vi "Layer2_ReceiveResponse.vi"(8 "Error In":errorcluster, 9 "PacketNum\nWaiting Ack":u16=9915, 10 "Expecting Response":bool, 11 "Serial Port to Use":refnum<visa-resource-name>="COM8") -> (0 "Layer2 Payload":string, 1 "No Errors":bool, 2 "Response Received":bool, 3 "Msg Acknowledged":bool, 4 "Error Out":errorcluster, 5 "Serial Port to Use (out)":refnum<visa-resource-name>)   [LabVIEW 2012]
uses:
  Arduino_Serial_GlobalConstants.vi
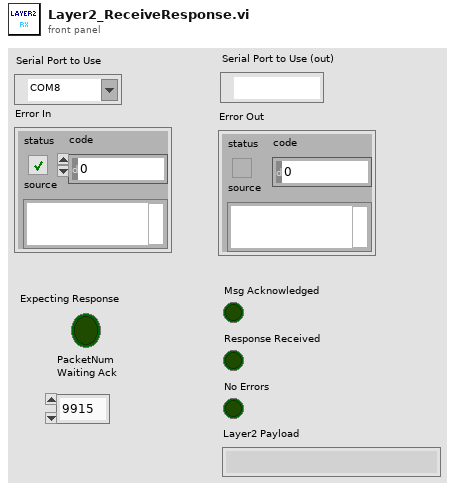
[diagram p1: front panel]
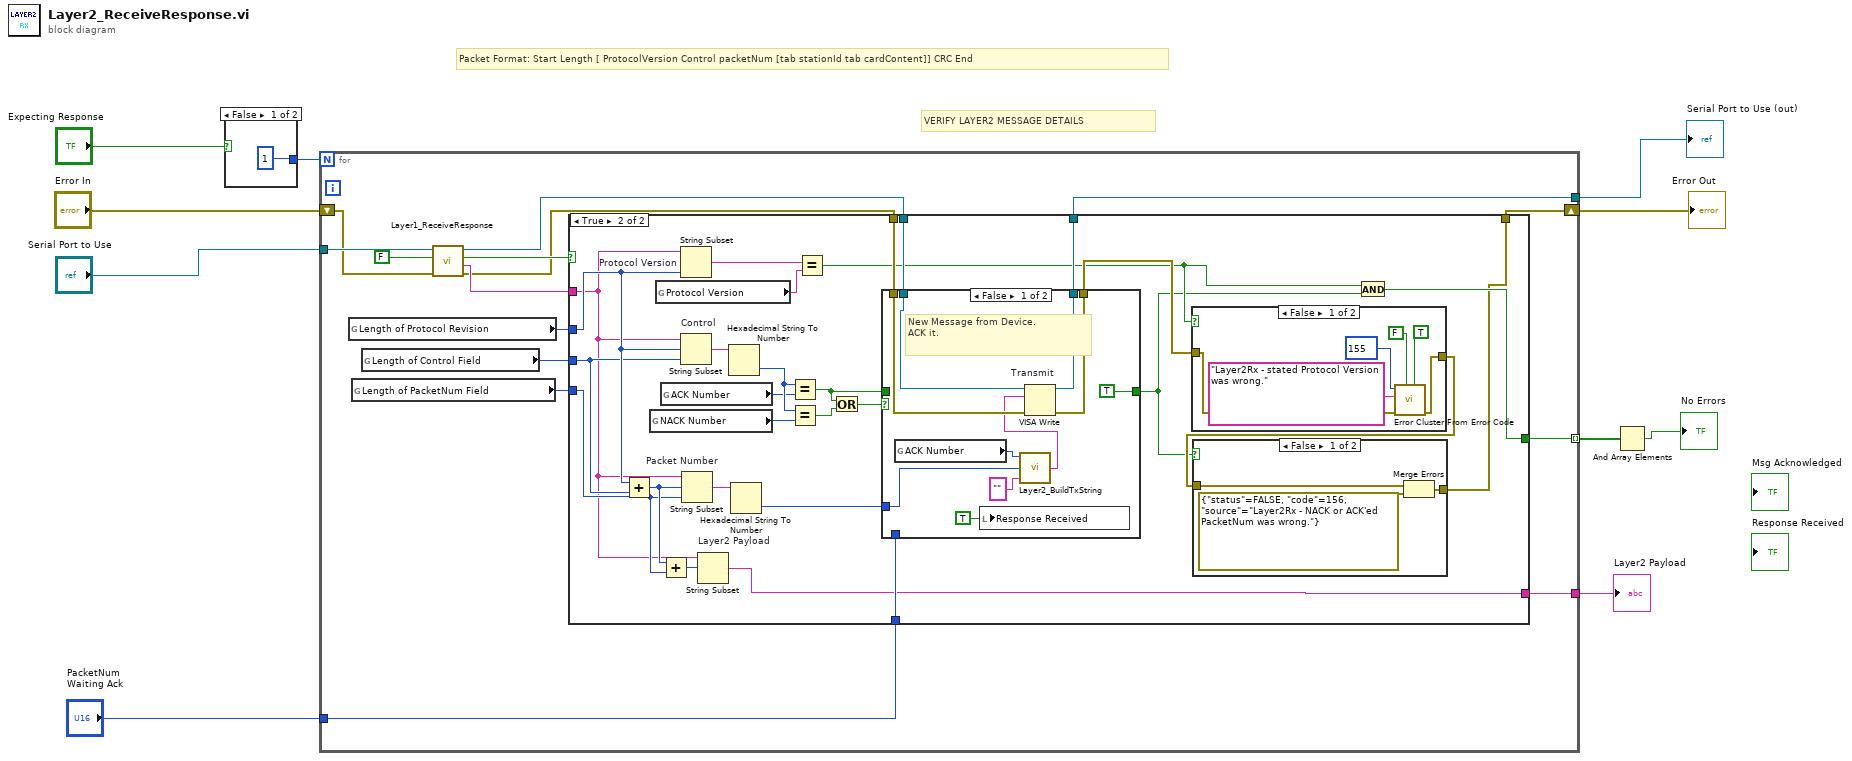
[diagram p0: block diagram]
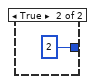
[diagram p2: hidden frame]
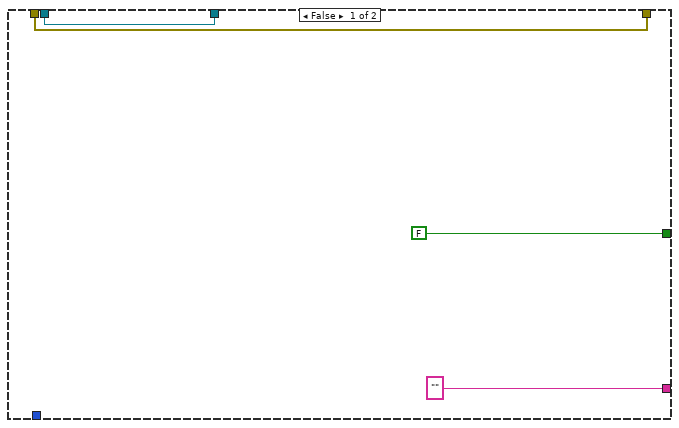
[diagram p3: hidden frame]
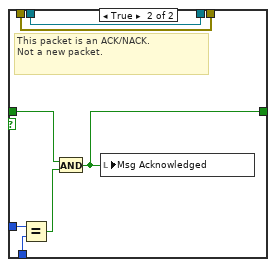
[diagram p6: hidden frame]
diagram:
  # "Packet Format: Start Length [ ProtocolVersion Control packetNum [tab stationId tab cardContent]] CRC End"
  # "VERIFY LAYER2 MESSAGE DETAILS"
  n1 = case shown="False" "Expecting Response" {
    tunnel: [1 ("Numeric") 2 ("Numeric")] -> w6
    frame False {
    }
    frame True {
    }
  }
  n2 = for {
    N: w6 -> [_]
    tunnel: "Serial Port to Use" -> [w27]
    tunnel: [w25] -> w8
    tunnel: [w24] -> w4 mode=indexing
    tunnel: "PacketNum\nWaiting Ack" -> [w23]
    shift-right: [w13] -> w1
    shift-left: "Error In" -> [w26]
    tunnel: [w14] -> w2
    n3 = global read "Arduino_Serial_GlobalConstants.vi" "Length of Protocol Revision"() -> (w20:i32)
    n4 = global read "Arduino_Serial_GlobalConstants.vi" "Length of PacketNum Field"() -> (w22:i32)
    n5 = global read "Arduino_Serial_GlobalConstants.vi" "Length of Control Field"() -> (w21:i32)
    n6 = call "Layer1_ReceiveResponse.vi"("Error In"=w26, "Close Port After?"=FALSE, "Serial Port to Use (In)"=w27) -> ("Error Out"=w15:errorcluster, "Layer1 Payload"=w18:string, "Layer 1 Valid Packet"=w17:bool, "Serial Port to Use (out)"=w16:refnum<visa-resource-name>)  [unwired: 3 in, 2 out]
    n7 = case shown="True" w17 {
      tunnel: [FALSE w37] -> w24
      tunnel: w18 -> [_ w51]
      tunnel: ["" ("read buffer") w38] -> w25
      tunnel: w23 -> [_ w41]
      tunnel: w22 -> [_ w53]
      tunnel: w21 -> [_ w56]
      tunnel: w20 -> [_ w57]
      tunnel: w15 -> [w28 w44]
      tunnel: w16 -> [w29 w43]
      tunnel: [w29 w42] -> w14
      tunnel: [w28 w34] -> w13
      frame False {
      }
      frame True {
        n8 = Add(x=w57, y=w56) -> (x+y=w54:i32)
        n9 = global read "Arduino_Serial_GlobalConstants.vi" "NACK Number"() -> (w47:i32)
        n10 = global read "Arduino_Serial_GlobalConstants.vi" "Protocol Version"() -> (w58:string)
        n11 = global read "Arduino_Serial_GlobalConstants.vi" "ACK Number"() -> (w48:i32)
        n12 = Add(x=w54, y=w53) -> (x+y=w52:i32)
        n13 = String Subset "Protocol Version"(string=w51, length (rest)=w57) -> (substring=w59:string)  [unwired: 1 in]
        n14 = String Subset "Control"(string=w51, offset (0)=w57, length (rest)=w56) -> (substring=w50:string)
        n15 = String Subset "Packet Number"(string=w51, offset (0)=w54, length (rest)=w53) -> (substring=w55:string)
        n16 = String Subset "Layer2 Payload"(string=w51, offset (0)=w52) -> (substring=w38:string)  [unwired: 1 in]
        n17 = Hexadecimal String To Number(string=w50) -> (number=w49:u32)  [unwired: 2 in, 1 out]
        n18 = Hexadecimal String To Number(string=w55) -> (number=w40:u32)  [unwired: 2 in, 1 out]
        n19 = Equal?(x=w49, y=w48) -> (x = y?=w39:bool)
        n20 = Equal?(x=w49, y=w47) -> (x = y?=w46:bool)
        n21 = Equal?(x=w59, y=w58) -> (x = y?=w35:bool)
        n22 = Or(x=w39, y=w46) -> (x .or. y?=w45:bool)
        n23 = case shown="False" w45 {
          tunnel: w44 -> [w74 w86]
          tunnel: w43 -> [w75 w87]
          tunnel: [w73 w87] -> w42
          tunnel: [w72 w86] -> w36
          tunnel: w41 -> [_ w85]
          tunnel: w40 -> [w78 w84]
          tunnel: [TRUE w81] -> w32
          tunnel: w39 -> [_ w82]
          frame False {
            # "New Message from Device.\nACK it."
            n24 = global read "Arduino_Serial_GlobalConstants.vi" "ACK Number"() -> (w76:i32)
            n25 = local write "Response Received"(TRUE ("Response Received")) -> ()
            n26 = call "Layer2_BuildTxString.vi"("Message"="", "PacketNum"=w78, "Control"=w76) -> ("Write Buffer"=w71:string)
            n27 = VISA Write "Transmit"(VISA resource name=w75, write buffer=w71, error in (no error)=w74) -> (VISA resource name out=w73:refnum<visa-resource-name>, error out=w72:errorcluster)  [unwired: 1 out]
          }
          frame True {
            # "This packet is an ACK/NACK.\nNot a new packet."
            n28 = Equal?(x=w84, y=w85) -> (x = y?=w83:bool)
            n29 = And(x=w82, y=w83) -> (x .and. y?=w81:bool)
            n30 = local write "Msg Acknowledged"(w81) -> ()
          }
        }
        n31 = case shown="False" w35 {
          tunnel: w36 -> [w69 w70]
          tunnel: [w68 w70] -> w33
          frame False {
            n32 = call <vilib>:"Error Cluster From Error Code.vi"("is warning? (False)"=TRUE, "show call chain? (False)"=FALSE, "error in (no error)"=w69, "error message (\"\")"="Layer2Rx - stated Protocol Version was wrong." ("source"), "error code (0)"=155 ("code")) -> ("error out"=w68:errorcluster)  [unwired: 4 in]
          }
          frame True {
          }
        }
        n33 = case shown="False" w32 {
          tunnel: w33 -> [w61 w63]
          tunnel: [w62 w63] -> w34
          frame False {
            n34 = Merge Errors(w61, errorcluster {"status"=FALSE, "code"=156, "source"="Layer2Rx - NACK or ACK'ed PacketNum was wrong."} ("error in")) -> (w62:errorcluster)
          }
          frame True {
          }
        }
        n35 = And(x=w35, y=w32) -> (x .and. y?=w37:bool)
      }
    }
  }
  "Layer2 Payload" <- w8
  "Error Out" <- w1
  "Serial Port to Use (out)" <- w2
  n36 = And Array Elements(Boolean array=w4) -> (logical AND=→"No Errors":bool)
